vi "PH_Beckhoff_PP_PU.handle PSU AIs.vi"(0 "i ref in":refnum<vi>, 2 "Analog Inputs":T1, 3 "Changed analog Inputs":i32[](array[numeric]), 5 "error in":errorcluster) -> (14 "i ref out":refnum<vi>, 19 "error out":errorcluster)   [LabVIEW 2014, in "PH_Beckhoff_PP_PU.lvlib"]
uses:
  PH_Beckhoff_PP_PU.lvlib
  PH_Beckhoff/PH_Beckhoff.Analog Inputs.ctl
  PH_Beckhoff/PH_Beckhoff.Scaling Type.ctl
  PH_Beckhoff/PH_Beckhoff.lvlib
  PH_Common/PH_Common.lvlib
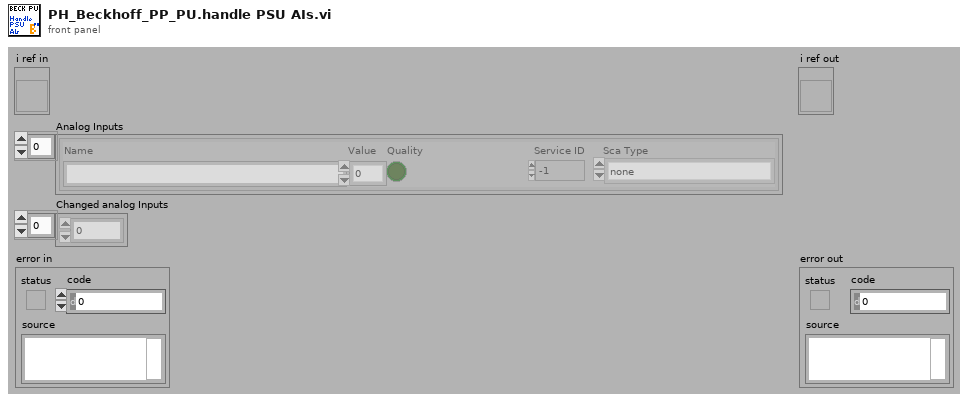
[diagram p1: front panel]
types:
  T1 = typedef "PH_Beckhoff.lvlib/PH_Beckhoff.Analog Inputs.ctl" = cluster{"Name":string, "Value":u32, "Quality":bool, "Service ID":i32, "Sca Type":T2}[]
  T2 = typedef "PH_Beckhoff.lvlib/PH_Beckhoff.Scaling Type.ctl" = enum16{"none", "0 ... 15 Bit -> 0 ... 5", "0 ... 15 Bit -> 0 ... 10", "0 ... 15 Bit -> 0 ... 25", "0 ... 15 Bit -> 4 ... 20", "0 ... 15 Bit -> 0 ... 1", "0 ... 15 Bit -> 0 ... 20000", "0 ... 15 Bit -> 0 ... 24000"}
  T3 = typedef "PH_Beckhoff_PP_PU.lvlib/PH_Beckhoff_PP_PU.i attribute.ctl" = cluster{"HV Meas":cluster{"Input GUI Ref":refnum<vi>, "Voltage Service ID":i32, "Voltage [V]":dbl, "Quality":bool, "# in Data":i32}[], "Trigger":cluster{"Status":cluster{"GUI Ref":refnum<vi>, "Status Service ID":i32, "Status":T4}, "last shot:":cluster{"GUI Ref":refnum<vi>, "Service ID":i32, "Time":string}, "DIs":cluster{"triggered":cluster{"GUI Ref":refnum<vi>, "# in Data":i32}, "fired":cluster{"GUI Ref":refnum<vi>, "# in Data":i32}}, "GUI Ref Indicator":refnum<vi>}[], "RR":cluster{"Status":cluster{"GUI Ref":refnum<vi>, "Status Service ID":i32, "Status":T4}, "DIs":cluster{"closed":cluster{"GUI Ref":refnum<vi>, "# in Data":i32}, "open":cluster{"GUI Ref":refnum<vi>, "# in Data":i32}}, "Close":cluster{"GUI Ref":refnum<vi>, "# in Data":i32}, "GUI Ref Indicator":refnum<vi>}[], "Igni":cluster{"Status":cluster{"GUI Ref":refnum<vi>, "Status Service ID":i32, "Status":T4}, "DIs":cluster{"heating on":cluster{"GUI Ref":refnum<vi>, "# in Data":i32}, "water on":cluster{"GUI Ref":refnum<vi>, "# in Data":i32}}, "Device on":cluster{"GUI Ref":refnum<vi>, "# in Data":i32}, "GUI Ref Indicator":refnum<vi>}[], "PSU":cluster{"Status":cluster{"GUI Ref":refnum<vi>, "Status Service ID":i32, "Status":T4}, "Limit Service ID":i32, "DIs":cluster{"inhibit":cluster{"GUI Ref":refnum<vi>, "# in Data":i32}, "end of charge":cluster{"GUI Ref":refnum<vi>, "# in Data":i32}, "HV on":cluster{"GUI Ref":refnum<vi>, "# in Data":i32}, "overtemp":cluster{"GUI Ref":refnum<vi>, "# in Data":i32}, "interlock":cluster{"GUI Ref":refnum<vi>, "# in Data":i32}, "load fault":cluster{"GUI Ref":refnum<vi>, "# in Data":i32}, "sum fault":cluster{"GUI Ref":refnum<vi>, "# in Data":i32}, "HV off":cluster{"GUI Ref":refnum<vi>, "# in Data":i32}, "DC ok":cluster{"GUI Ref":refnum<vi>, "# in Data":i32}}, "AIs":cluster{"voltage":cluster{"GUI Ref":refnum<vi>, "# in Data":i32}, "current":cluster{"GUI Ref":refnum<vi>, "# in Data":i32}}, "DAs":cluster{"inhibit":cluster{"GUI Ref":refnum<vi>, "# in Data":i32}, "interlock":cluster{"GUI Ref":refnum<vi>, "# in Data":i32}, "HV on":cluster{"GUI Ref":refnum<vi>, "# in Data":i32}, "Reset":cluster{"GUI Ref":refnum<vi>, "# in Data":i32}}, "AAs":cluster{"Voltage to set":cluster{"GUI Ref":refnum<vi>, "# in Data":i32}}, "GUI Ref Indicator":refnum<vi>}[], "reconfigured":cluster{"?":bool, "GUI Ref":refnum<vi>}, "PU Rack Type":T5, "HV Meas Info":T6, "PSU Info":T7}
  T4 = typedef "PH_StatusHandler.lvlib/PH_StatusHandler.Status.ctl" = i16
  T5 = typedef "PH_Beckhoff_PP_PU.lvlib/PH_Beckhoff_PP_PU.PU Rack Type.ctl" = enum16{"no Info", "PA 19mm", "PA 45mm", "MA PU 1 and 2", "MA PU 3 and 4", "MA PU 5 and 6", "MA FR and PILC"}
  T6 = typedef "PH_Beckhoff_PP_PU.lvlib/PH_Beckhoff_PP_PU.HV Meas Info.ctl" = cluster{"Period Time [s]":dbl, "Subtractor 1 [Hz]":dbl, "Devider 1 [Hz/kV]":dbl, "Subtractor 2 [Hz]":dbl, "Devider 2 [Hz/kV]":dbl}
  T7 = typedef "PH_Beckhoff_PP_PU.lvlib/PH_Beckhoff_PP_PU.PSU Info.ctl" = cluster{"Limits 1 [V]":cluster{"Lower":dbl, "Upper":dbl}, "Limits 2 [V]":cluster{"Lower":dbl, "Upper":dbl}}
  T8 = cluster{"Status":cluster{"GUI Ref":refnum<vi>, "Status Service ID":i32, "Status":T4}, "Limit Service ID":i32, "DIs":cluster{"inhibit":cluster{"GUI Ref":refnum<vi>, "# in Data":i32}, "end of charge":cluster{"GUI Ref":refnum<vi>, "# in Data":i32}, "HV on":cluster{"GUI Ref":refnum<vi>, "# in Data":i32}, "overtemp":cluster{"GUI Ref":refnum<vi>, "# in Data":i32}, "interlock":cluster{"GUI Ref":refnum<vi>, "# in Data":i32}, "load fault":cluster{"GUI Ref":refnum<vi>, "# in Data":i32}, "sum fault":cluster{"GUI Ref":refnum<vi>, "# in Data":i32}, "HV off":cluster{"GUI Ref":refnum<vi>, "# in Data":i32}, "DC ok":cluster{"GUI Ref":refnum<vi>, "# in Data":i32}}, "AIs":cluster{"voltage":cluster{"GUI Ref":refnum<vi>, "# in Data":i32}, "current":cluster{"GUI Ref":refnum<vi>, "# in Data":i32}}, "DAs":cluster{"inhibit":cluster{"GUI Ref":refnum<vi>, "# in Data":i32}, "interlock":cluster{"GUI Ref":refnum<vi>, "# in Data":i32}, "HV on":cluster{"GUI Ref":refnum<vi>, "# in Data":i32}, "Reset":cluster{"GUI Ref":refnum<vi>, "# in Data":i32}}, "AAs":cluster{"Voltage to set":cluster{"GUI Ref":refnum<vi>, "# in Data":i32}}, "GUI Ref Indicator":refnum<vi>}[]
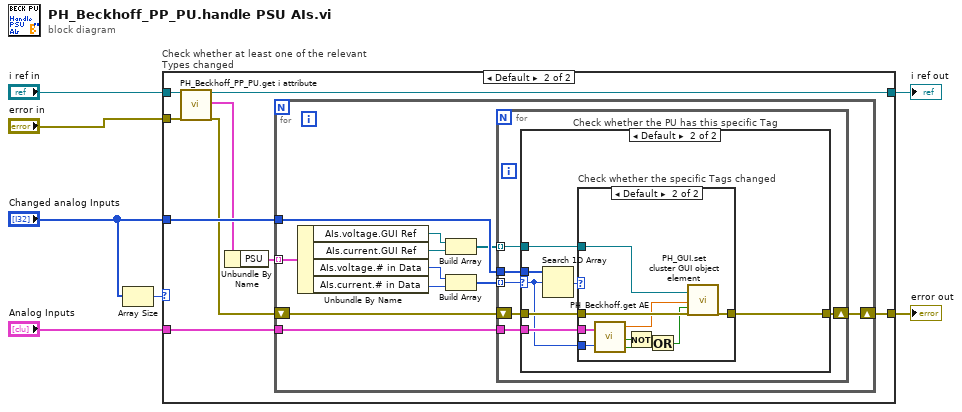
[diagram p0: block diagram]
diagram:
  n1 = Array Size(array="Changed analog Inputs") -> (size(s)=w3:i32)
  n2 = case "Check whether at least one of the relevant Types changed" shown="Default" w3 {
    tunnel: "error in" -> [w9 w16]
    tunnel: [w9 w18] -> w1
    tunnel: "Changed analog Inputs" -> [_ w17]
    tunnel: [w8 w14] -> w2
    tunnel: "i ref in" -> [w8 w13]
    tunnel: "Analog Inputs" -> [_ w10]
    frame 0 {
    }
    frame Default {
      n3 = call "PH_Beckhoff_PP_PU.get i attribute.vi"("i ref in"=w13, "error in (no error)"=w16) -> ("i ref out"=w14:refnum<vi>, "i attribute"=w12:T3, "error out"=w15:errorcluster)  [unwired: 15 in]
      n4 = Unbundle By Name(w12) -> ("PSU"=w11:T8)
      n5 = for {
        tunnel: w10 -> [w19]
        tunnel: w17 -> [w28]
        shift-right: [w29] -> w18
        shift-left: w15 -> [w27]
        tunnel: w11 -> [w26] mode=indexing
        n6 = Unbundle By Name(w26) -> ("AIs.voltage.GUI Ref"=w24:refnum<vi>, "AIs.current.GUI Ref"=w25:refnum<vi>, "AIs.voltage.# in Data"=w22:i32, "AIs.current.# in Data"=w23:i32)
        n7 = Build Array(w24, w25) -> (w21:refnum<vi>[])
        n8 = Build Array(w22, w23) -> (w20:i32[])
        n9 = for {
          tunnel: w19 -> [w33]
          tunnel: w21 -> [w32] mode=indexing
          tunnel: w20 -> [w31] mode=indexing
          tunnel: w28 -> [w30]
          shift-right: [w34] -> w29
          shift-left: w27 -> [w35]
          n10 = case "Check whether the PU has this specific Tag" shown="Default" w31 {
            selector: w31 -> [_ w39]
            tunnel: w35 -> [w36 w43]
            tunnel: [w36 w42] -> w34
            tunnel: w33 -> [_ w41]
            tunnel: w32 -> [_ w40]
            tunnel: w30 -> [_ w38]
            frame -1 {
            }
            frame Default {
              n11 = Search 1D Array(1D array=w38, element=w39) -> (index of element=w37:i32)  [unwired: 1 in]
              n12 = case "Check whether the specific Tags changed" shown="Default" w37 {
                tunnel: w43 -> [w44 w49]
                tunnel: [w44 w48] -> w42
                tunnel: w41 -> [_ w50]
                tunnel: w40 -> [_ w47]
                tunnel: w39 -> [_ w51]
                frame -1 {
                }
                frame Default {
                  n13 = call "PH_Beckhoff.get AE.vi"("Analog Inputs"=w50, "index of element"=w51) -> ("DIM value"=w46:dbl, "Quality"=w53:bool, "Tag not found"=w54:bool)
                  n14 = Not(x=w53) -> (.not. x?=w52:bool)
                  n15 = Or(x=w52, y=w54) -> (x .or. y?=w45:bool)
                  n16 = call "PH_GUI.set cluster GUI object element.vi"("Ctl Refnum"=w47, "Value"=w46, "Blinking? (false)"=w45, "error in"=w49) -> ("error out"=w48:errorcluster)  [unwired: 15 in]
                }
              }
            }
          }
        }
      }
    }
  }
  "i ref out" <- w2
  "error out" <- w1
